vi "VelocityAndFreq.vi"(7 "Divs":i32=128, 10 "CurrenMeters":cluster{"Array":timestamp[], "Array":dbl[]}[](array[cluster]), 11 "Specs_time":cluster{"Waveform":waveform(dbl), timestamp}[](array[cluster])) -> (3 "3D Plot lvclass Array out":refnum<class "3D Plot Datatype.lvclass">[](array[class]))   [LabVIEW 2016]
uses:
  <vilib>/Math Plots/3D Math Plots/3D Surface/3D Surface XCtrl/3D Surface.xctl
  <vilib>/Math Plots/3D Math Plots/3D Plot/3D Plot Datatype/3D Plot Datatype.lvclass
  <vilib>/Analysis/1siggen.llb/Ramp Pattern by Samples.vi
  <vilib>/Math Plots/3D Math Plots/3D Surface/3D Surface Datatype/Public/Plot Helper (Vector).vi
  <vilib>/Analysis/NI_AALBase.lvlib
  <vilib>/Math Plots/3D Math Plots/3D Surface/3D Surface Datatype/3D Surface Datatype.lvclass
panel:
  out "Superficie":refnum<class "3D Plot Datatype.lvclass">[](xcontrol)
  out "Specs":dbl[][](graph)
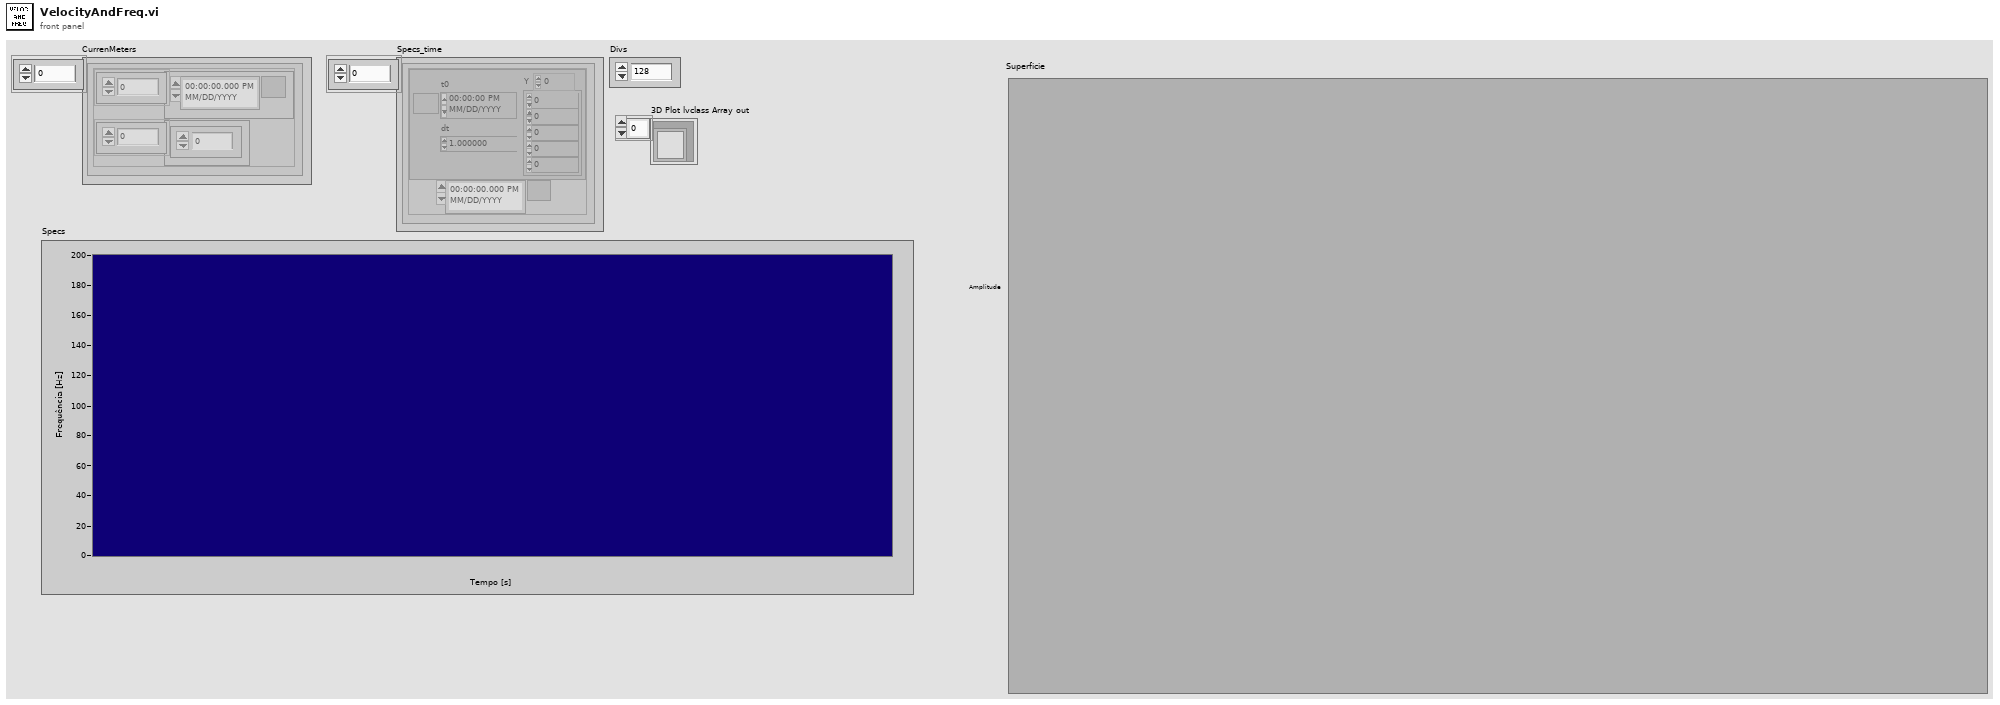
[diagram p1: front panel]
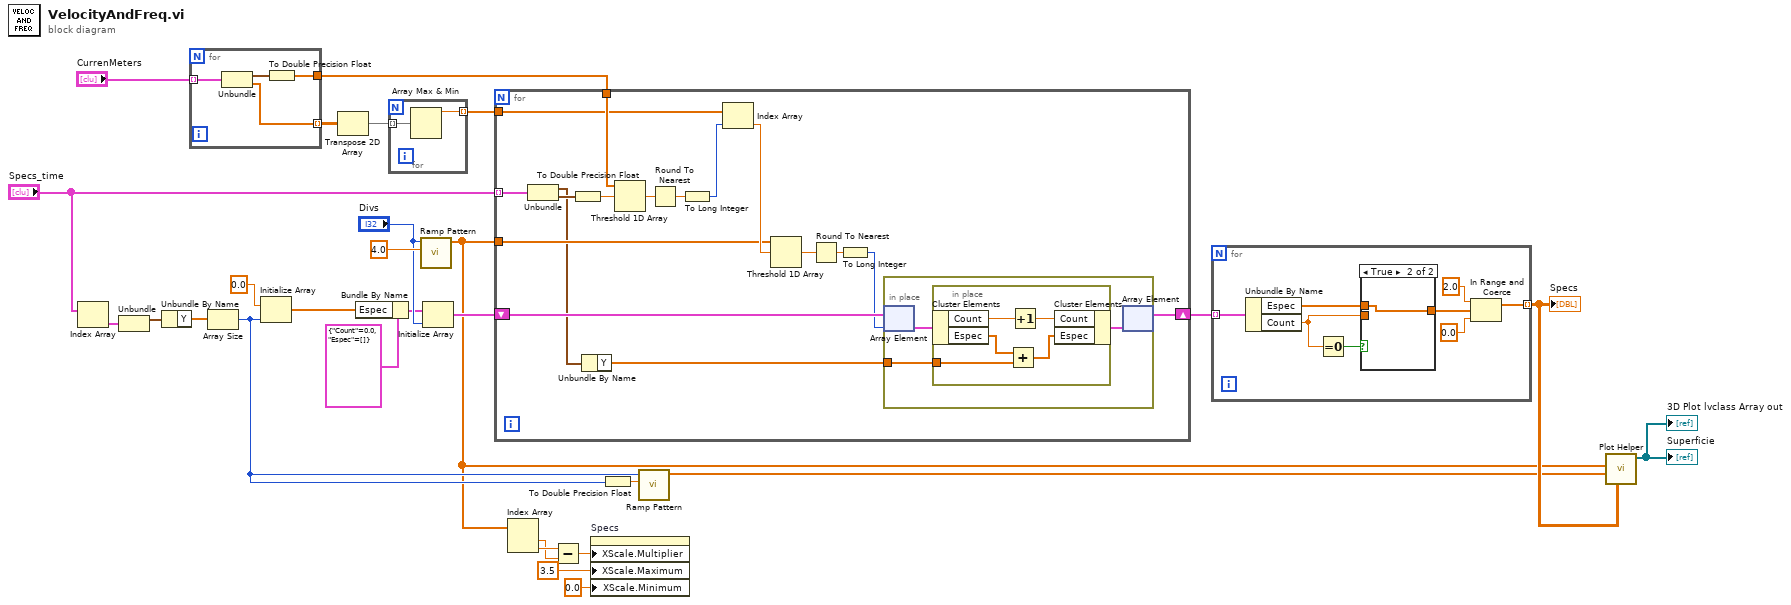
[diagram p0: block diagram]
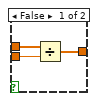
[diagram p2: hidden frame]
diagram:
  n1 = Index Array(array="Specs_time") -> (element=w25:cluster{"Waveform":waveform(dbl), timestamp})  [unwired: 1 in]
  n2 = Unbundle(w25) -> ("Waveform"=w24:waveform(dbl))  [unwired: 1 out]
  n3 = Unbundle By Name(w24) -> ("Y"=w23:dbl[])
  n4 = for {
    tunnel: "CurrenMeters" -> [w32] mode=indexing
    tunnel: [w30] -> w17
    tunnel: [w29] -> w16 mode=indexing
    n5 = Unbundle(w32) -> ("Array"=w31:timestamp[], "Array"=w29:dbl[])
    n6 = To Double Precision Float(number=w31) -> (double precision float=w30:dbl[])
  }
  n7 = Array Size(array=w23) -> (size(s)=w4:i32)
  n8 = Initialize Array(0.0 ("end"), w4) -> (w20:dbl[])
  n9 = Transpose 2D Array(2D array=w16) -> (transposed array=w15:dbl[][])
  n10 = Bundle By Name(cluster=cluster{"Count":dbl, "Espec":dbl[]} {"Count"=0.0, "Espec"=[]}, "Espec"=w20) -> (w19:cluster{"Count":dbl, "Espec":dbl[]})
  n11 = for {
    tunnel: w15 -> [w34] mode=indexing
    tunnel: [w33] -> w14 mode=indexing
    n12 = Array Max & Min(array=w34) -> (max value=w33:dbl)  [unwired: 3 out]
  }
  n13 = call-poly <vilib>:"Ramp Pattern.vi"("end"=4.0, "samples"="Divs") -> ("Ramp Pattern"=w1:dbl[])  [unwired: 8 in, 1 out]
  n14 = Initialize Array(w19, "Divs") -> (w13:cluster{"Count":dbl, "Espec":dbl[]}[])
  n15 = for {
    tunnel: "Specs_time" -> [w51] mode=indexing
    tunnel: w17 -> [w49]
    tunnel: w14 -> [w45]
    tunnel: w1 -> [w42]
    shift-right: [w36] -> w12
    shift-left: w13 -> [w41]
    n16 = Unbundle(w51) -> ("Waveform"=w38:waveform(dbl), w50:timestamp)
    n17 = To Double Precision Float(number=w50) -> (double precision float=w48:dbl)
    n18 = Unbundle By Name(w38) -> ("Y"=w37:dbl[])
    n19 = Threshold 1D Array(2:w48, 3:w49) -> (0:w47:dbl)  [unwired: 1 in]
    n20 = Round To Nearest(number=w47) -> (nearest integer value=w46:dbl)
    n21 = To Long Integer(number=w46) -> (32bit integer=w35:i32)
    n22 = Index Array(array=w45, index=w35) -> (element=w43:dbl)
    n23 = Threshold 1D Array(2:w43, 3:w42) -> (0:w44:dbl)  [unwired: 1 in]
    n24 = Round To Nearest(number=w44) -> (nearest integer value=w40:dbl)
    n25 = To Long Integer(number=w40) -> (32bit integer=w39:i32)
    n26 = in-place {
      in-place-border: w37 -> [w53]
      n27 = in-place-array #1(w41, w39) -> (w54:cluster{"Count":dbl, "Espec":dbl[]})
      n28 = in-place {
        in-place-border: w53 -> [w56]
        n29 = in-place-cluster #2(w54) -> ("Count"=w59:dbl, "Espec"=w57:dbl[])
        n30 = Add(x=w57, y=w56) -> (x+y=w55:dbl[])
        n31 = Increment(x=w59) -> (x+1=w58:dbl)
        n32 = in-place-cluster #2("Count"=w58, "Espec"=w55) -> (w52:cluster{"Count":dbl, "Espec":dbl[]})
      }
      n33 = in-place-array #1(w52) -> (w36:cluster{"Count":dbl, "Espec":dbl[]}[])  [unwired: 1 out]
    }
  }
  n34 = Index Array(array=w1) -> (element #1=w10:dbl, element #2=w11:dbl)  [unwired: 2 in]
  n35 = Subtract(x=w11, y=w10) -> (x-y=w9:dbl)
  n36 = property on="Specs" class="IntGraph (strict)"("XScale.Multiplier"=w9, "XScale.Maximum"=3.5 ("X Scale.Range:Maximum"), "XScale.Minimum"=0.0 ("X Scale.Range:Minimum")) -> ()  [unwired: 2 in, 2 out]
  n37 = To Double Precision Float(number=w4) -> (double precision float=w3:dbl)
  n38 = call-poly <vilib>:"Ramp Pattern.vi"("end"=w3, "samples"=w4) -> ("Ramp Pattern"=w2:dbl[])  [unwired: 8 in, 1 out]
  n39 = for {
    tunnel: w12 -> [w67] mode=indexing
    tunnel: [w60] -> w5 mode=indexing
    n40 = Unbundle By Name(w67) -> ("Espec"=w65:dbl[], "Count"=w64:dbl)
    n41 = Equal To 0?(x=w64) -> (x = 0?=w66:bool)
    n42 = case shown="True" w66 {
      tunnel: w65 -> [w70 w71]
      tunnel: w64 -> [w69 _]
      tunnel: [w68 w71] -> w63
      frame False {
        n43 = Divide(x=w70, y=w69) -> (x/y=w68:dbl[])
      }
      frame True {
      }
    }
    n44 = In Range and Coerce(upper limit=2.0 ("end"), x=w63, lower limit=0.0 ("end")) -> (coerced(x)=w60:dbl[])  [unwired: 1 out]
  }
  "Specs" <- w5
  n45 = call-poly <vilib>:"Plot Helper.vi"("z matrix"=w5, "y vector"=w2, "x vector"=w1) -> ("3D Plot lvclass Array out"=→"Superficie" →"3D Plot lvclass Array out":refnum<class "3D Plot Datatype.lvclass">[])  [unwired: 3 in, 5 out]
